vi "Generate Digital Pulse with control on RPM.vi"() -> ()   [LabVIEW 2019, in "Part of Main VIs.lvlib" / "Tachometer Library.lvlib"]
uses:
  Tachometer Library.lvlib
  <extravilib>/ChannelInstances/Tag-dbl/Read With Abort.vi
  <extravilib>/ChannelInstances/Tag-dbl/Write With Abort.vi
  <extravilib>/ChannelInstances/Tag-dbl/Instantiate.vi
  <vilib>/DAQmx/create/channels.llb/DAQmx Create Channel (CO-Pulse Generation-Time).vi
  <vilib>/DAQmx/configure/timing.llb/DAQmx Timing (Implicit).vi
  <extravilib>/ChannelInstances/Tag-dbl/EndpointRead.vi
  <extravilib>/ChannelInstances/Tag-dbl/Endpoint.vi
  Tachometer VI.lvlib
  <resource>/objmgr/daqmx.rc
  <extravilib>/ChannelInstances/Tag-dbl.lvlib
panel:
  out "# waiting":dbl
  out "latest notification":dbl
  out "notification":dbl
  out "created new?":bool
  out "cache entry size (in bytes)":i32
  out "total cache size (in bytes)":i32
  out "# of cache levels":i32
  out "# of logical processors per core":i32
  out "# of cores per package":i32
  out "# of packages":i32
  out "# of logical processors":i32
  out "CO.CtrTimebaseSrc":tag
  out "CO.Pulse.Term":tag
  out "CO.Pulse.HighTime":dbl
  out "CO.Pulse.LowTime":dbl
  out "Frequency":dbl
  out "Period":dbl
  in  "RPM":dbl=1000.0
  out "Low Time":dbl
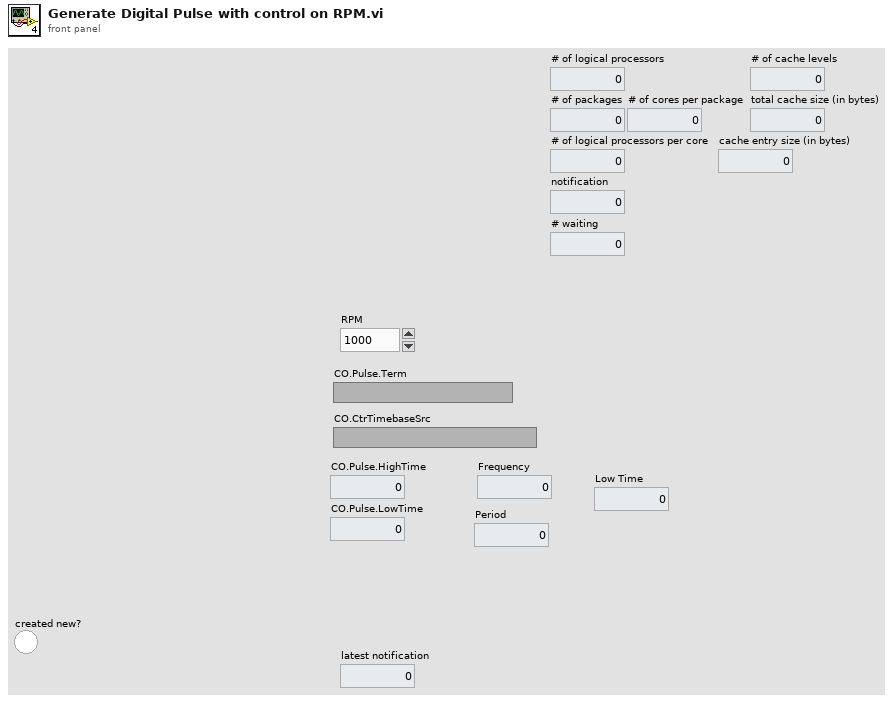
[diagram p1: front panel]
types:
  T1 = typedef "Tag-dbl.lvlib/))Channel.ctl" = refnum<queue>
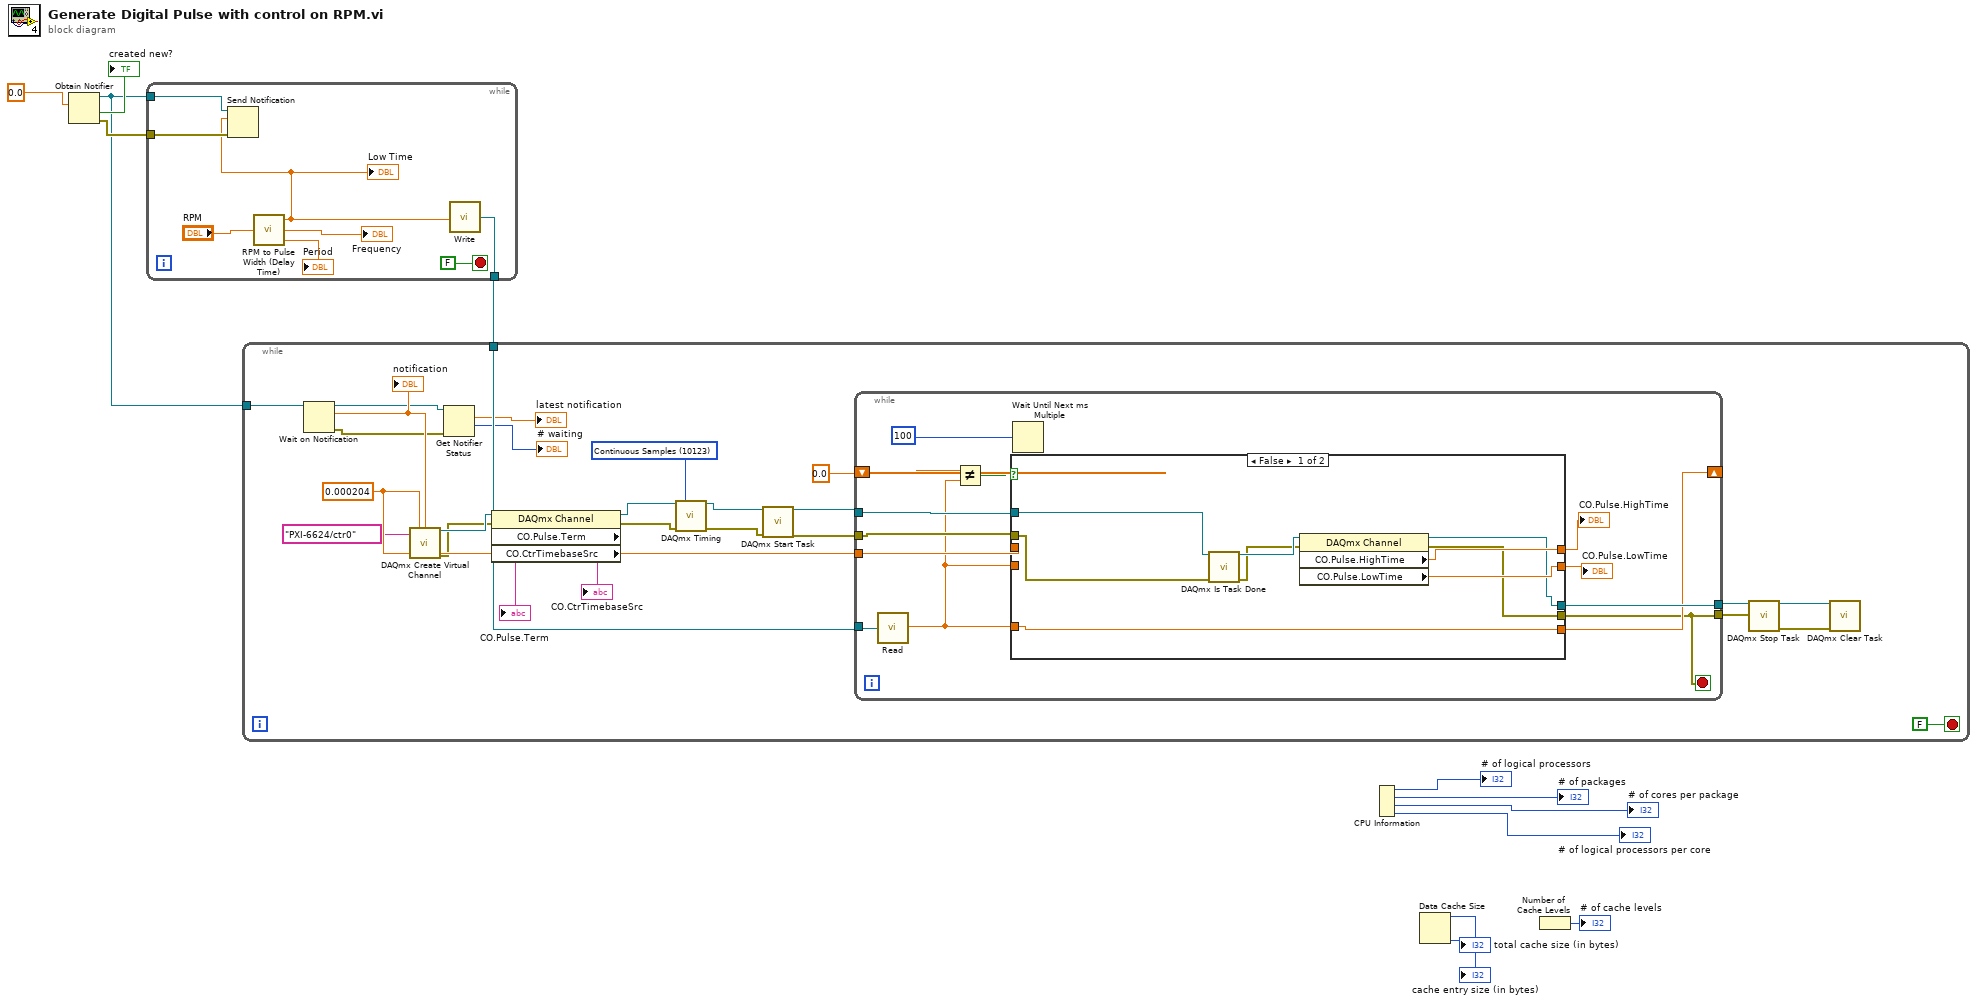
[diagram p0: block diagram]
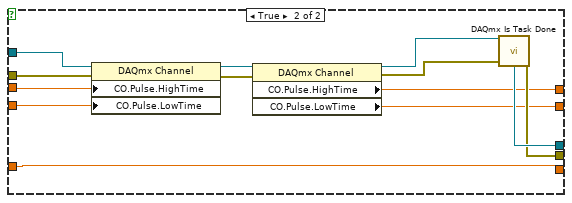
[diagram p2: hidden frame]
diagram:
  n1 = Obtain Notifier(notification data type=0.0) -> (notifier out=w1:refnum<notifier>, created new?=→"created new?":bool, error out=w4:errorcluster)  [unwired: 3 in]
  n2 = while {
    tunnel: [w19] -> w12
    tunnel: w1 -> [w15]
    tunnel: w4 -> [w14]
    stop <- FALSE stop-if-true
    n3 = call "RPM to Pulse Width (Delay Time).vi"("RPM"="RPM") -> ("Period"=→"Period":dbl, "Frequency"=→"Frequency":dbl, "Low Time"=w13:dbl)  [unwired: 2 in]
    "Low Time" <- w13
    n4 = Send Notification(notification=w13, notifier=w15, error in (no error)=w14) -> ()  [unwired: 2 out]
    n5 = call <extravilib>:"Write.vi"("element"=w13) -> ("channel"=w19:T1)  [unwired: 1 out]
  }
  n6 = while {
    tunnel: w12 -> [w46]
    tunnel: w1 -> [w26]
    stop <- FALSE stop-if-true
    w41 = 0.000204 ("high time")
    w40 = 10123 items=["Finite Samples"=10178, "Continuous Samples"=10123, "Hardware Timed Single Point"=12522] ("sample mode")
    n7 = Wait on Notification(notifier=w26) -> (notifier out=w24:refnum<notifier>, notification=w25:dbl, error out=w23:errorcluster)  [unwired: 3 in, 1 out]
    "notification" <- w25
    n8 = call-poly <vilib>:"DAQmx Create Virtual Channel.vi"("high time"=w41, "low time"=w25, "counter"=tag "PXI-6624/ctr0") -> ("task out"=w38:refnum<k21>, "error out"=w37:errorcluster)  [unwired: 11 in]
    n9 = Get Notifier Status(notifier=w24, error in (no error)=w23) -> (current notification=→"latest notification":dbl, # waiting=→"# waiting":i32)  [unwired: 3 out]
    n10 = property class="DAQmx Channel"(reference=w38, error in=w37) -> (reference out=w33:refnum<k21>, error out=w32:errorcluster, "CO.Pulse.Term"=→"CO.Pulse.Term":tag, "CO.CtrTimebaseSrc"=→"CO.CtrTimebaseSrc":tag)
    n11 = call-poly <vilib>:"DAQmx Timing.vi"("task/channels in"=w33, "sample mode"=w40, "error in"=w32) -> ("task out"=w31:refnum<k21>, "error out"=w30:errorcluster)  [unwired: 11 in]
    n12 = call <vilib>:"DAQmx Start Task.vi"("task/channels in"=w31, "error in"=w30) -> ("task out"=w29:refnum<k21>, "error out"=w28:errorcluster)  [unwired: 12 in]
    n13 = while {
      tunnel: w28 -> [w56]
      tunnel: w29 -> [w57]
      shift-right: [w51] -> _
      shift-left: 0.0 ("element") -> [w52]
      tunnel: w41 -> [w50]
      tunnel: [w55] -> w43
      tunnel: [w48] -> w42
      tunnel: w46 -> [w49]
      stop <- w48 stop-if-true
      n14 = call <extravilib>:"Read.vi"("channel"=w49) -> ("element"=w47:dbl)  [unwired: 1 in, 1 out]
      n15 = Not Equal?(x=w52, y=w47) -> (x != y?=w58:bool)
      n16 = case shown="False" w58 {
        tunnel: w57 -> [w68 w81]
        tunnel: w56 -> [w67 w80]
        tunnel: w50 -> [_ w77]
        tunnel: [w62 w79] -> w55
        tunnel: [w61 w78] -> w48
        tunnel: [w64 w74] -> w54
        tunnel: [w63 w73] -> w53
        tunnel: w47 -> [w60 w69]
        tunnel: [w60 w69] -> w51
        tunnel: w47 -> [_ w70]
        frame False {
          n17 = call <vilib>:"DAQmx Is Task Done.vi"("task/channels in"=w68, "error in"=w67) -> ("task out"=w66:refnum<k21>, "error out"=w65:errorcluster)  [unwired: 11 in, 1 out]
          n18 = property class="DAQmx Channel"(reference=w66, error in=w65) -> (reference out=w62:refnum<k21>, error out=w61:errorcluster, "CO.Pulse.HighTime"=w64:dbl, "CO.Pulse.LowTime"=w63:dbl)
        }
        frame True {
          n19 = property class="DAQmx Channel"(reference=w81, error in=w80, "CO.Pulse.HighTime"=w77, "CO.Pulse.LowTime"=w70) -> (reference out=w76:refnum<k21>, error out=w75:errorcluster)
          n20 = property class="DAQmx Channel"(reference=w76, error in=w75) -> (reference out=w72:refnum<k21>, error out=w71:errorcluster, "CO.Pulse.HighTime"=w74:dbl, "CO.Pulse.LowTime"=w73:dbl)
          n21 = call <vilib>:"DAQmx Is Task Done.vi"("task/channels in"=w72, "error in"=w71) -> ("task out"=w79:refnum<k21>, "error out"=w78:errorcluster)  [unwired: 11 in, 1 out]
        }
      }
      "CO.Pulse.HighTime" <- w54
      "CO.Pulse.LowTime" <- w53
      n22 = Wait Until Next ms Multiple(millisecond multiple=100) -> ()  [unwired: 1 out]
    }
    n23 = call <vilib>:"DAQmx Stop Task.vi"("task/channels in"=w43, "error in"=w42) -> ("task out"=w45:refnum<k21>, "error out"=w44:errorcluster)  [unwired: 12 in]
    n24 = call <vilib>:"DAQmx Clear Task.vi"("task in"=w45, "error in"=w44) -> ()  [unwired: 13 in, 1 out]
  }
  n25 = CPU Information() -> (4:→"# of logical processors":i32, 5:→"# of packages":i32, 6:→"# of cores per package":i32, 7:→"# of logical processors per core":i32)
  n26 = Data Cache Size() -> (4:→"total cache size (in bytes)":i32, 7:→"cache entry size (in bytes)":i32)  [unwired: 1 in]
  n27 = Number of Cache Levels() -> (→"# of cache levels":i32)
